vi "参数设置对画框.vi"(8 "时间等比采样":u16=10, 9 "单次采样量":u16=500, 10 "整点定时时间":T1, 11 "留样模式":enum16{"定时采样", "外控采样", "时间等比", "流量等比", "液位等比"}(ring)=enum."液位等比") -> ()   [LabVIEW 2016, in "超标留样集成.lvlib" / "ESTD1200.lvlib"]
uses:
  ESTD1200.lvlib
  <vilib>/Utility/config.llb/NI_LVConfig.lvlib
  <vilib>/Plasmionique/MB Master/MB Master.lvlib
panel:
  in  "内部参数":bool
  in  "关闭":bool
  in  "打开串口":bool
  in  "释放串口":bool
  # "只在停止时切换有效"
  # "默认：500ml（5-1000）ml （只在停止时写有效）"
  # "默认：10min（2-9999）min （只在停止时写有效）"
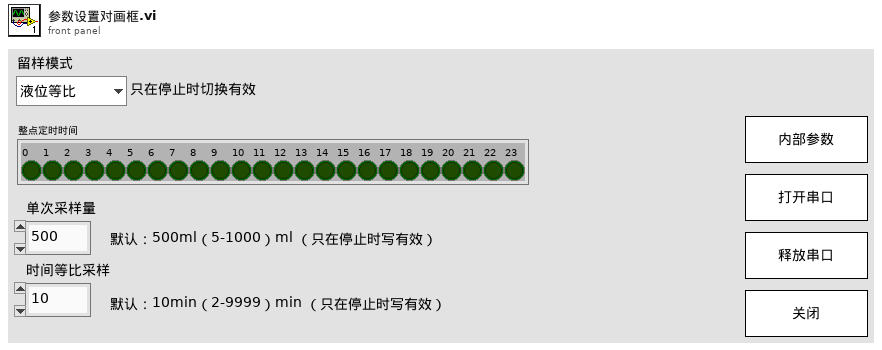
[diagram p1: front panel]
types:
  T1 = cluster{"0":bool, "1":bool, "2":bool, "3":bool, "4":bool, "5":bool, "6":bool, "7":bool, "8":bool, "9":bool, "10":bool, "11":bool, "12":bool, "13":bool, "14":bool, "15":bool, "16":bool, "17":bool, "18":bool, "19":bool, "20":bool, "21":bool, "22":bool, "23":bool}
  T2 = typedef "队列data.ctl" = cluster{"命令":string, "data":cluster{"站号":u16, "控制命令":u16[]}}
  T3 = cluster{"命令":string, "data":cluster{"站号":u16, "控制命令":u16[]}}
  T4 = typedef "NI_LVConfig.lvlib/Config Data RefNum.ctl" = refnum<k1>
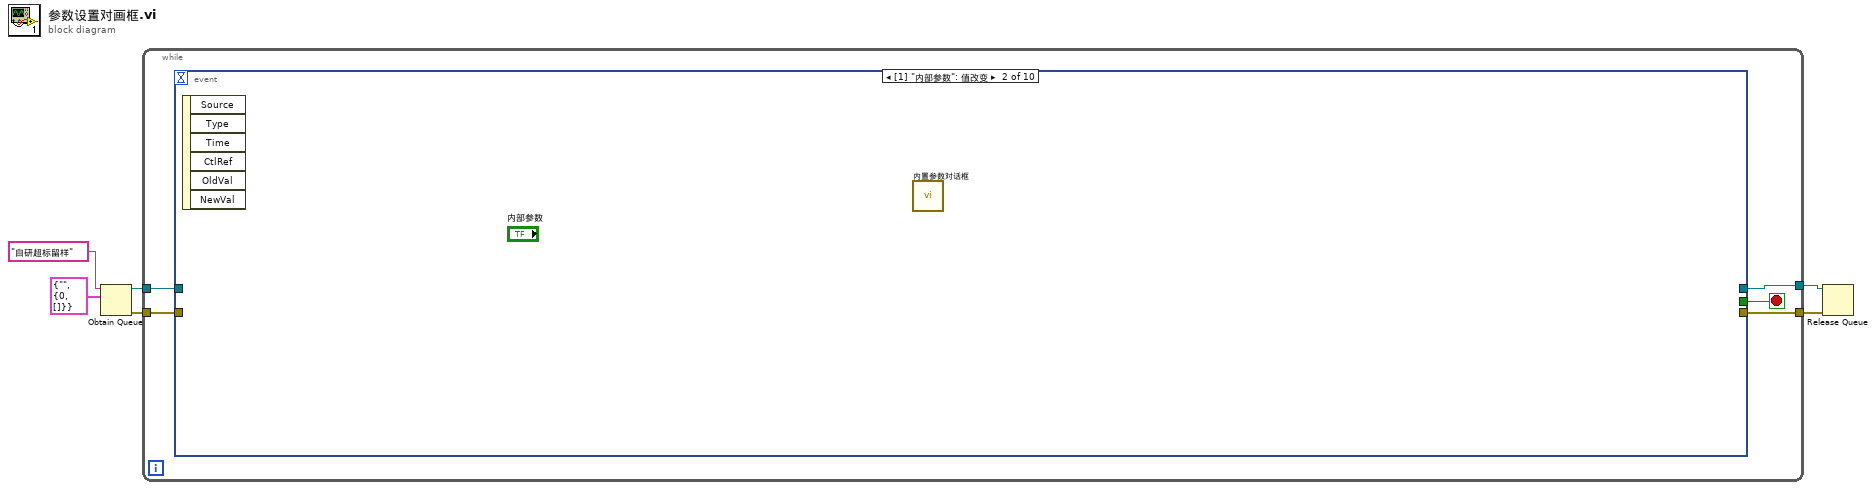
[diagram p0: block diagram]
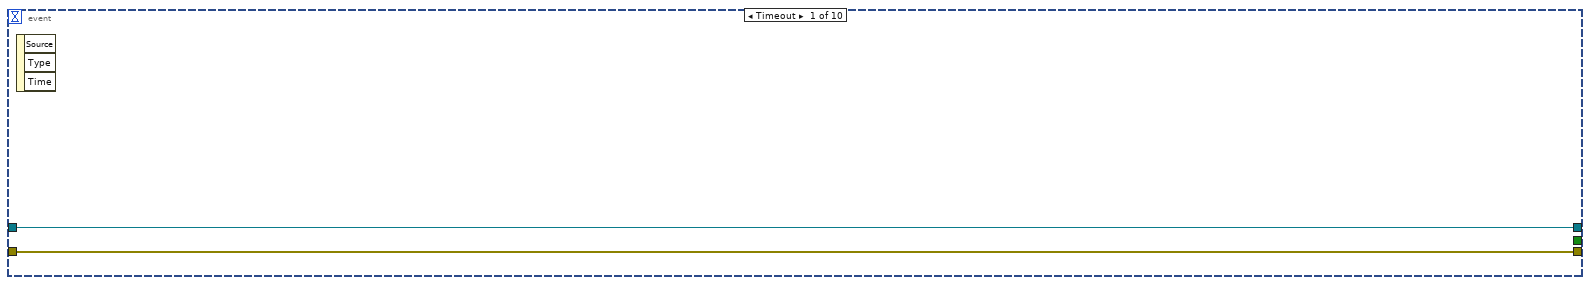
[diagram p2: hidden frame]
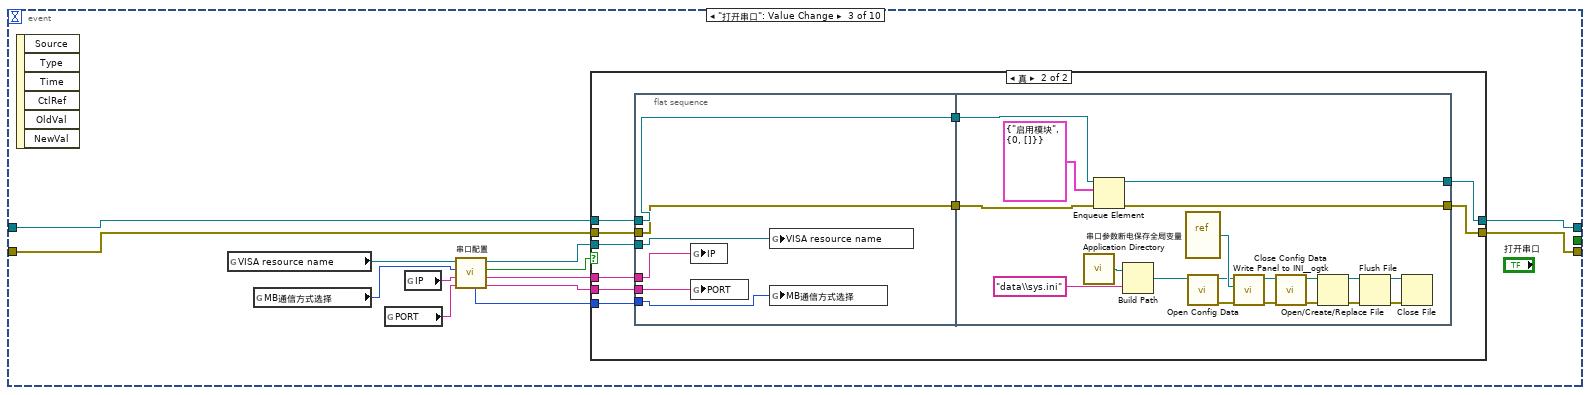
[diagram p3: hidden frame]
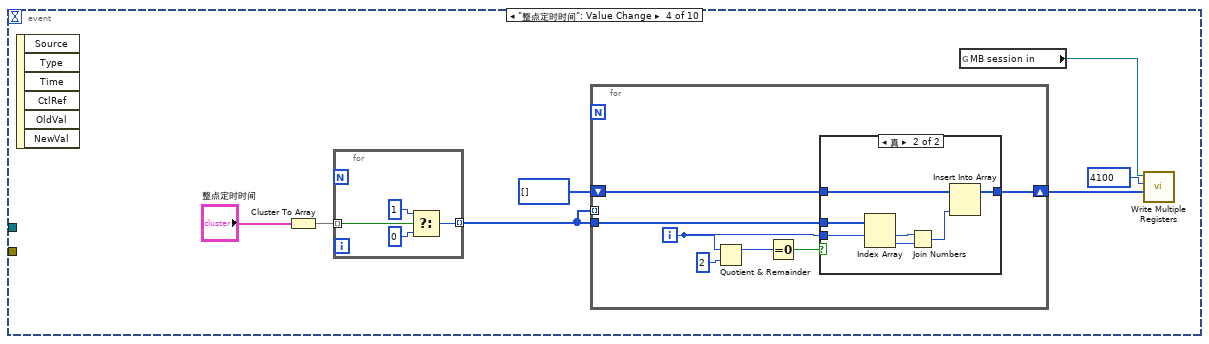
[diagram p5: hidden frame]
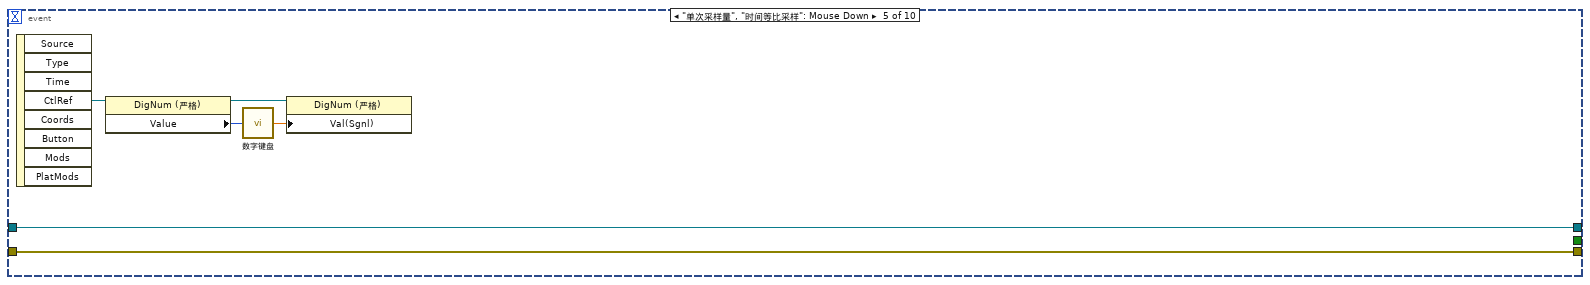
[diagram p7: hidden frame]
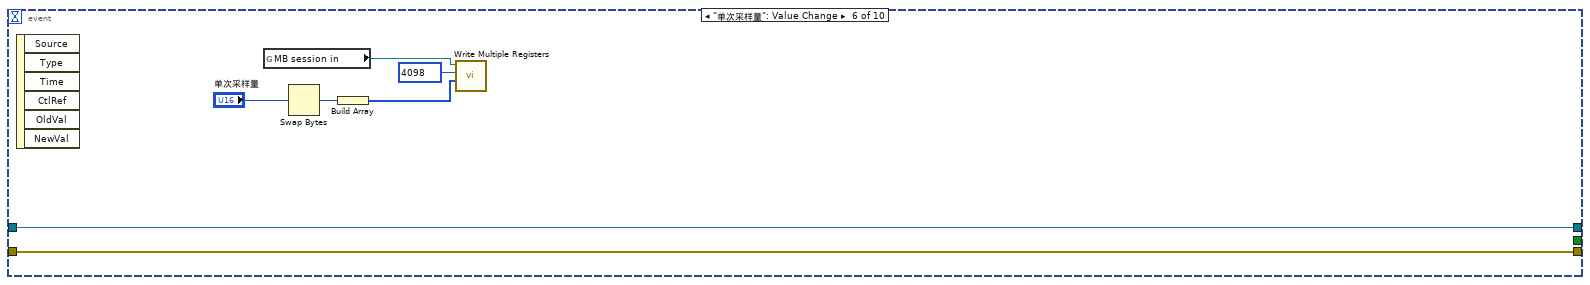
[diagram p8: hidden frame]
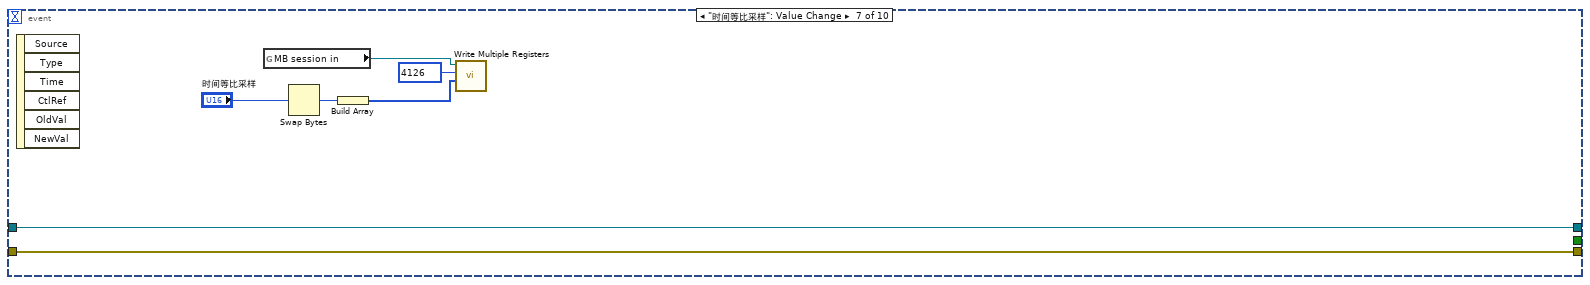
[diagram p9: hidden frame]
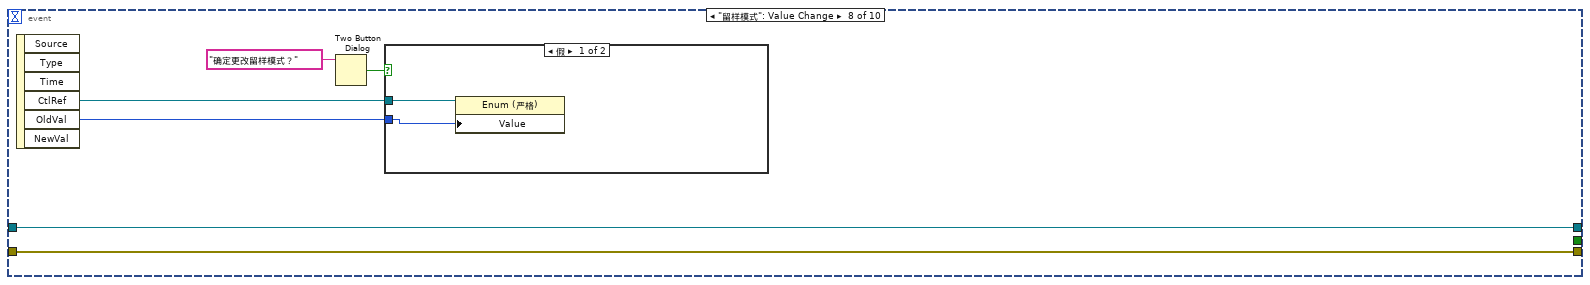
[diagram p10: hidden frame]
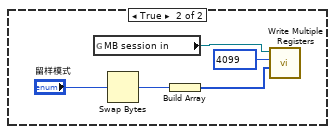
[diagram p11: hidden frame]
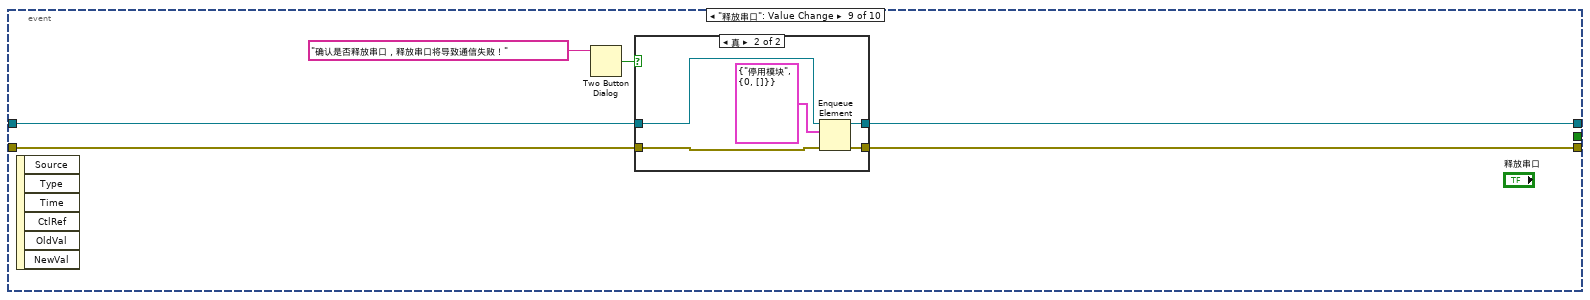
[diagram p12: hidden frame]
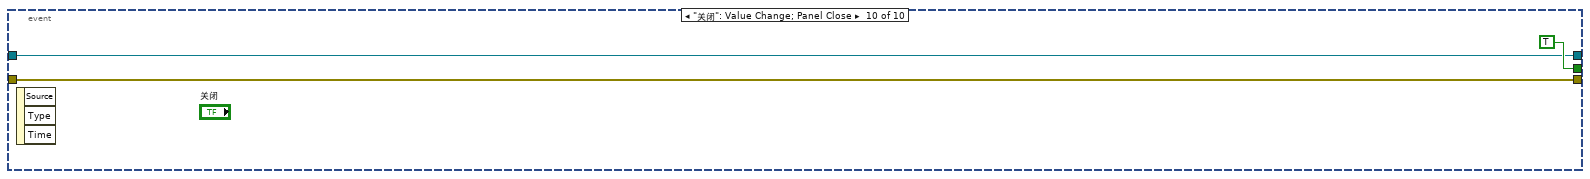
[diagram p14: hidden frame]
diagram:
  n1 = Obtain Queue(name (unnamed)="自研超标留样" ("名称（未命名）"), element data type=T2 {"命令"="", "data"={"站号"=0, "控制命令"=[]}}) -> (queue out=w2:refnum<queue>, error out=w1:errorcluster)  [unwired: 3 in, 1 out]
  n2 = while {
    tunnel: w2 -> [w11]
    tunnel: w1 -> [w10]
    tunnel: [w9] -> w6
    tunnel: [w8] -> w5
    stop <- w7 stop-if-true
    n3 = event shown="[1] \"内部参数\": 值改变" {
      selector: _ -> [_ _ _ _ _ _ _ _ _ _]
      dyn-events: _ -> [_ _ _ _ _ _ _ _ _ _]
      timeout: _ -> [_ _ _ _ _ _ _ _ _ _]
      tunnel: w11 -> [w13 _ w17 _ w91 w102 w109 w111 w126 w137]
      tunnel: w10 -> [w12 _ w16 _ w90 w101 w108 w110 w125 w136]
      tunnel: [w13 _ w15 _ w91 w102 w109 w111 w124 w137] -> w9
      tunnel: [w12 _ w14 _ w90 w101 w108 w110 w123 w136] -> w8
      tunnel: [_ _ _ _ _ _ _ _ _ TRUE] -> w7
      event Timeout {
        n4 = event-data() -> ()  [unwired: 1 in, 3 out]
      }
      event "内部参数": Value Change {
        n5 = event-data() -> ()  [unwired: 1 in, 6 out]
        n6 = call "内置参数对话框.vi"() -> ()  [unwired: 12 in]
      }
      event "打开串口": Value Change {
        n7 = event-data() -> ()  [unwired: 1 in, 6 out]
        n8 = global read "串口参数断电保存全局变量.vi" "VISA resource name"() -> (w19:refnum<visa-resource-name>)
        n9 = global read "串口参数断电保存全局变量.vi" "MB通信方式选择"() -> (w18:enum16{"串口", "TCP"})
        n10 = global read "串口参数断电保存全局变量.vi" "PORT"() -> (w21:string)
        n11 = global read "串口参数断电保存全局变量.vi" "IP"() -> (w20:string)
        n12 = call "串口配置.vi"("PORT"=w21, "IP"=w20, "MB通信方式选择"=w18, "请选择串口:"=w19) -> ("PORT 2"=w25:string, "IP 2"=w24:string, "确认 2"=w22:bool, "VISA资源名称 2"=w23:refnum<visa-resource-name>, "MB通信方式选择 2"=w26:enum16{"串口", "TCP"})  [unwired: 3 in]
        n13 = case shown="真" w22 {
          tunnel: w23 -> [_ w38]
          tunnel: w24 -> [_ w37]
          tunnel: w25 -> [_ w36]
          tunnel: w26 -> [_ w35]
          tunnel: w17 -> [w28 w34]
          tunnel: w16 -> [w27 w32]
          tunnel: [w28 w30] -> w15
          tunnel: [w27 w29] -> w14
          frame False {
          }
          frame True {
            n14 = flat-sequence {
              tunnel: w38 -> [w44]
              tunnel: w37 -> [w43]
              tunnel: w36 -> [w42]
              tunnel: w35 -> [w41]
              tunnel: w34 -> [w40]
              tunnel: [w40] -> w33
              tunnel: w32 -> [w39]
              tunnel: [w39] -> w31
              tunnel: w33 -> [w49]
              tunnel: w31 -> [w48]
              tunnel: [w47] -> w30
              tunnel: [w46] -> w29
              frame #0 {
                n15 = global write "串口参数断电保存全局变量.vi" "IP"(w43) -> ()
                n16 = global write "串口参数断电保存全局变量.vi" "PORT"(w42) -> ()
                n17 = global write "串口参数断电保存全局变量.vi" "VISA resource name"(w44) -> ()
                n18 = global write "串口参数断电保存全局变量.vi" "MB通信方式选择"(w41) -> ()
              }
              frame #1 {
                n19 = call <vilib>:"Application Directory.vi"() -> ("Application Directory"=w51:path)
                n20 = Enqueue Element(queue=w49, element=T3 {"命令"="启用模块", "data"={"站号"=0, "控制命令"=[]}} ("元素"), error in (no error)=w48) -> (queue out=w47:refnum<queue>, error out=w46:errorcluster)  [unwired: 1 in, 1 out]
                n21 = Build Path(base path=w51, name or relative path="data\\sys.ini" ("名称或相对路径")) -> (appended path=w52:path)
                n22 = vi-ref "串口参数断电保存全局变量.vi"() -> (w54:refnum<vi>)
                n23 = call <vilib>:"Open Config Data.vi"("configuration file path"=w52) -> ("error out"=w56:errorcluster, "refnum"=w53:T4)  [unwired: 8 in, 1 out]
                n24 = call <userlib>:"Write Panel to INI__ogtk.vi"("error in (no error)"=w56, "VI ref"=w54, "refnum"=w53) -> ("error out"=w57:errorcluster, "refnum out"=w55:T4)  [unwired: 7 in]
                n25 = call <vilib>:"Close Config Data.vi"("error in (no error)"=w57, "refnum"=w55) -> ("error out"=w62:errorcluster, "file path"=w63:path)  [unwired: 8 in]
                n26 = Open/Create/Replace File(file path (use dialog)=w63, error in=w62) -> (refnum out=w59:refnum<file>, error out=w58:errorcluster)  [unwired: 4 in, 1 out]
                n27 = Flush File(refnum=w59, error in=w58) -> (refnum out=w60:refnum<file>, error out=w61:errorcluster)
                n28 = Close File(refnum=w60, error in=w61) -> ()  [unwired: 2 out]
              }
            }
          }
        }
      }
      event "整点定时时间": Value Change {
        n29 = event-data() -> ()  [unwired: 1 in, 6 out]
        n30 = Cluster To Array(cluster="整点定时时间") -> (array=w67:bool[])
        n31 = for {
          tunnel: w67 -> [w89] mode=indexing
          tunnel: [w86] -> w65 mode=indexing
          n32 = Select(t=u8 1, s=w89, f=u8 0) -> (s? t:f=w86:u8)
        }
        n33 = for {
          tunnel: w65 -> [_] mode=indexing
          tunnel: w65 -> [w74]
          shift-right: [w71] -> w64
          shift-left: u16[] [] -> [w72]
          i -> [w73]
          n34 = Quotient & Remainder(x=w73, y=2) -> (x-y*floor(x/y)=w76:i32)  [unwired: 1 out]
          n35 = Equal To 0?(x=w76) -> (x = 0?=w75:bool)
          n36 = case shown="真" w75 {
            tunnel: w74 -> [_ w85]
            tunnel: w73 -> [_ w84]
            tunnel: w72 -> [w78 w81]
            tunnel: [w78 w79] -> w71
            frame False {
            }
            frame True {
              n37 = Index Array(array=w85, index #1=w84) -> (element #1=w83:u8, element #2=w82:u8)  [unwired: 1 in]
              n38 = Join Numbers(hi=w83, lo=w82) -> ((hi.lo)=w80:u16)
              n39 = Insert Into Array(array=w81, new element=w80) -> (w79:u16[])  [unwired: 1 in]
            }
          }
        }
        n40 = global read "超标留样全局.vi" "MB session in"() -> (w70:refnum<class "MB_Master.lvclass">)
        n41 = call <vilib>:"Write Multiple Registers.vi"("values"=w64, "starting address"=u16 4100, "MB session in"=w70) -> ()  [unwired: 7 in, 2 out]
      }
      event "单次采样量", "时间等比采样": Mouse Down {
        n42 = event-data() -> ("CtlRef"=w92:refnum<vi>)  [unwired: 1 in, 7 out]
        n43 = property class="DigNum (严格)"(reference=w92) -> (reference out=w95:refnum<vi>, "Value"=w94:u16)  [unwired: 1 in, 1 out]
        n44 = call "数字键盘.vi"("OldNumber"=w94) -> ("NewNumber"=w93:sgl)
        n45 = property class="DigNum (严格)"(reference=w95, "Val(Sgnl)"=w93) -> ()  [unwired: 1 in, 2 out]
      }
      event "单次采样量": Value Change {
        n46 = event-data() -> ()  [unwired: 1 in, 6 out]
        n47 = global read "超标留样全局.vi" "MB session in"() -> (w100:refnum<class "MB_Master.lvclass">)
        n48 = Swap Bytes(anything="单次采样量") -> (byte swapped=w97:u16)
        n49 = Build Array(w97) -> (w99:u16[])
        n50 = call <vilib>:"Write Multiple Registers.vi"("values"=w99, "starting address"=u16 4098, "MB session in"=w100) -> ()  [unwired: 7 in, 2 out]
      }
      event "时间等比采样": Value Change {
        n51 = event-data() -> ()  [unwired: 1 in, 6 out]
        n52 = global read "超标留样全局.vi" "MB session in"() -> (w104:refnum<class "MB_Master.lvclass">)
        n53 = Swap Bytes(anything="时间等比采样") -> (byte swapped=w106:u16)
        n54 = Build Array(w106) -> (w105:u16[])
        n55 = call <vilib>:"Write Multiple Registers.vi"("values"=w105, "starting address"=u16 4126, "MB session in"=w104) -> ()  [unwired: 7 in, 2 out]
      }
      event "留样模式": Value Change {
        n56 = event-data() -> ("CtlRef"=w113:refnum<vi>, "OldVal"=w112:enum16{"定时采样", "外控采样", "时间等比", "流量等比", "液位等比"})  [unwired: 1 in, 4 out]
        n57 = Two Button Dialog(message="确定更改留样模式？" ("消息")) -> (T button?=w114:bool)  [unwired: 2 in]
        n58 = case shown="假" w114 {
          tunnel: w112 -> [w116 _]
          tunnel: w113 -> [w117 _]
          frame False {
            n59 = property class="Enum (严格)"(reference=w117, "Value"=w116) -> ()  [unwired: 1 in, 2 out]
          }
          frame True {
            n60 = global read "超标留样全局.vi" "MB session in"() -> (w122:refnum<class "MB_Master.lvclass">)
            n61 = Swap Bytes(anything="留样模式") -> (byte swapped=w120:u16)
            n62 = Build Array(w120) -> (w121:u16[])
            n63 = call <vilib>:"Write Multiple Registers.vi"("values"=w121, "starting address"=u16 4099, "MB session in"=w122) -> ()  [unwired: 7 in, 2 out]
          }
        }
      }
      event "释放串口": Value Change {
        n64 = event-data() -> ()  [unwired: 1 in, 6 out]
        n65 = Two Button Dialog(message="确认是否释放串口，释放串口将导致通信失败！" ("消息")) -> (T button?=w127:bool)  [unwired: 2 in]
        n66 = case shown="真" w127 {
          tunnel: w126 -> [w130 w135]
          tunnel: w125 -> [w129 w134]
          tunnel: [w130 w133] -> w124
          tunnel: [w129 w132] -> w123
          frame False {
          }
          frame True {
            n67 = Enqueue Element(queue=w135, element=T3 {"命令"="停用模块", "data"={"站号"=0, "控制命令"=[]}} ("元素"), error in (no error)=w134) -> (queue out=w133:refnum<queue>, error out=w132:errorcluster)  [unwired: 1 in, 1 out]
          }
        }
      }
      event "关闭": Value Change; Panel Close {
        n68 = event-data() -> ()  [unwired: 1 in, 3 out]
      }
    }
  }
  n69 = Release Queue(queue=w6, error in (no error)=w5) -> ()  [unwired: 1 in, 3 out]
